vi "GEA2 Register for Events.vi"(0 "GEA2 Reference In":refnum<k24>, 11 "Error In":errorcluster) -> (4 "GEA2 Reference Out":refnum<k24>, 6 "Event Registration Refnum":refnum<event-registration>, 15 "Error Out":errorcluster)   [LabVIEW 2020, in "GEA2_Toolkit.lvlib"]
doc: "This VI registers for events such that any messages that appear on the GEA2 bus trigger an event in LabVIEW. This event can be wired into an event structure and the message can be handled."
uses:
  library/GEA2_Toolkit.lvlib
  C:/TechnologyLab/NI-2010/Drivers/GEA3 Toolkit/GEA3 DLL Source/GeaCommunication.dll
  GEA3 DLL Source/GeaCommunication.dll
  type defs/Data Out.ctl
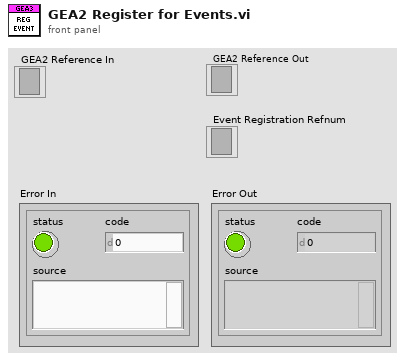
[diagram p1: front panel]
types:
  T1 = typedef "GEA2_Toolkit.lvlib/Data Out.ctl" = cluster{"Source":u8, "Destination":u8, "Command":u8, "Length":u8, "CRC":u16, "Message":string}
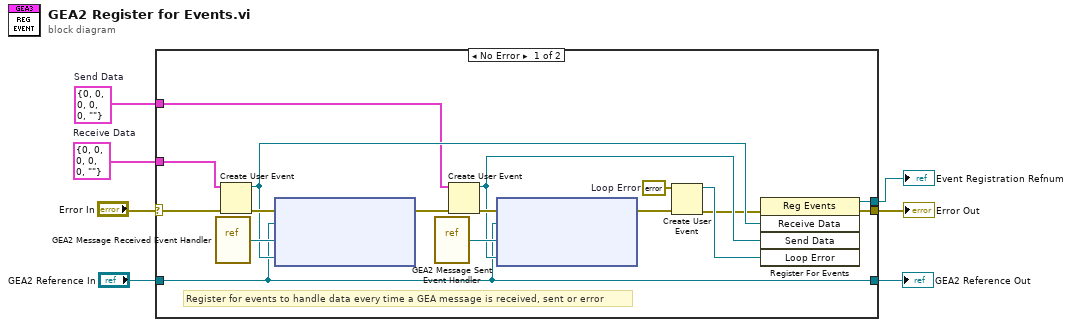
[diagram p0: block diagram]
diagram:
  w2 = T1 {"Source"=0, "Destination"=0, "Command"=0, "Length"=0, "CRC"=0, "Message"=""}  # Send Data
  w7 = T1 {"Source"=0, "Destination"=0, "Command"=0, "Length"=0, "CRC"=0, "Message"=""}  # Receive Data
  n1 = case shown="No Error" "Error In" {
    selector: "Error In" -> [w22 w26]
    tunnel: [w24 w26] -> w3
    tunnel: w7 -> [w17 _]
    tunnel: "GEA2 Reference In" -> [w10 w25]
    tunnel: [w10 w25] -> w6
    tunnel: w2 -> [w9 _]
    tunnel: [w8 _] -> w1
    frame No Error {
      w12 = errorcluster {"status"=FALSE, "code"=0, "source"=""}  # Loop Error
      # "Register for events to handle data every time a GEA message is received, sent or error"
      n2 = vi-ref "GEA2 Message Received Event Handler.vi"() -> (w21:refnum<vi>)
      n3 = Create User Event(user event datatype=w17, error in=w22) -> (user event=w20:refnum<user-event>, error out=w23:errorcluster)
      n4 = node(w23, w10, w21, w20) -> (w19:errorcluster)  [unwired: 1 in, 1 out]
      n5 = vi-ref "GEA2 Message Sent Event Handler.vi"() -> ("vi reference"=w16:refnum<vi>)
      n6 = Create User Event(user event datatype=w9, error in=w19) -> (user event=w15:refnum<user-event>, error out=w18:errorcluster)
      n7 = node(w18, w10, w16, w15) -> (w14:errorcluster)  [unwired: 1 in, 1 out]
      n8 = Create User Event(user event datatype=w12, error in=w14) -> (user event=w13:refnum<user-event>, error out=w11:errorcluster)
      n9 = register-events(error in=w11, w20, w15, w13) -> (reference out=w8:refnum<event-registration>, error out=w24:errorcluster)  [unwired: 1 in]
    }
    frame Error {
    }
  }
  "GEA2 Reference Out" <- w6
  "Error Out" <- w3
  "Event Registration Refnum" <- w1
